vi "MessageName.vi"() -> (2 "MessageName":string)   [LabVIEW 2020, in "StringData.lvlib"]
uses:
  StringData.lvlib
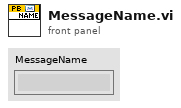
[diagram p1: front panel]
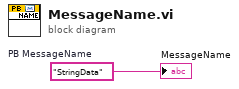
[diagram p0: block diagram]
diagram:
  w1 = "StringData"  # PB MessageName
  "MessageName" <- w1
